vi "VI-Fill Temp Event Cluster.vi"(0 "VI in":refnum<vi>, 2 "Components":T1, 9 "Names":string[](array[string]), 11 "error in (no error)":errorcluster) -> (4 "VI out":refnum<vi>, 15 "error out":errorcluster)   [LabVIEW 2015]
uses:
  VI-Reg Event Components.ctl
  <vilib>/Utility/miscctls.llb/LVPointTypeDef.ctl
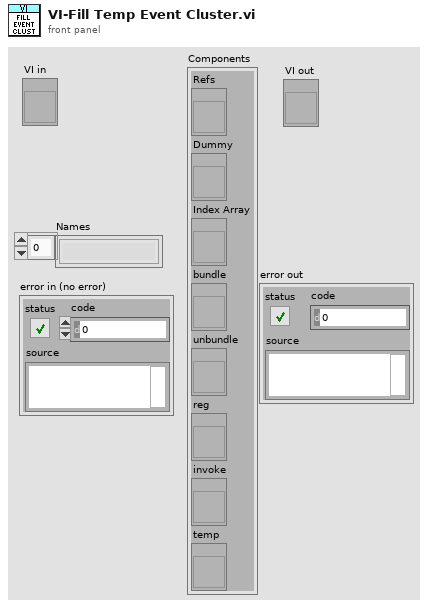
[diagram p1: front panel]
types:
  T1 = typedef "VI-Reg Event Components.ctl" = cluster{"Refs":refnum<vi>, "Dummy":refnum<vi>, "Index Array":refnum<vi>, "bundle":refnum<vi>, "unbundle":refnum<vi>, "reg":refnum<vi>, "invoke":refnum<vi>, "temp":refnum<vi>}
  T2 = typedef "LVPointTypeDef.ctl" = cluster{"Horizontal":i16, "Vertical":i16}
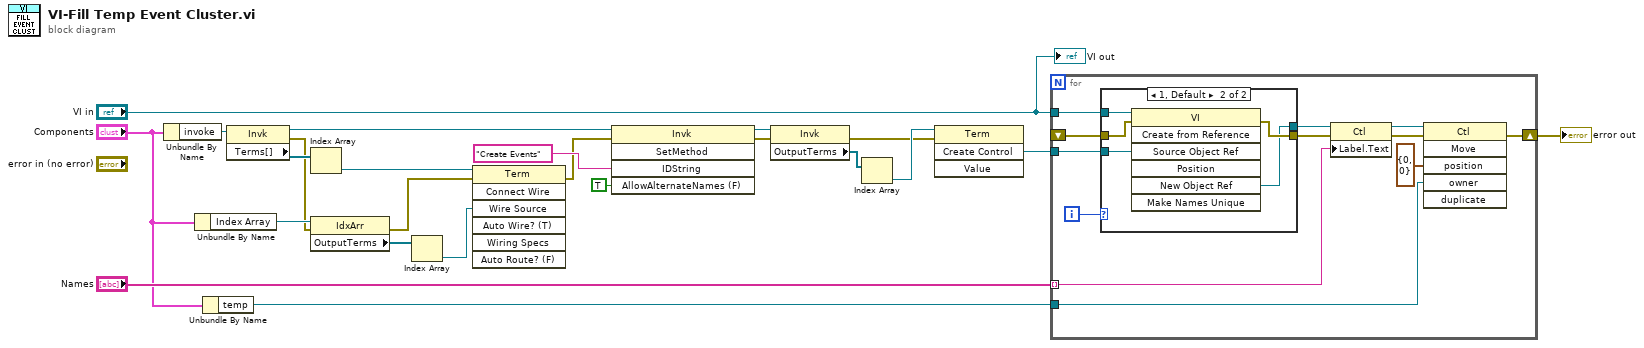
[diagram p0: block diagram]
diagram:
  n1 = Unbundle By Name("Components") -> ("invoke"=w1:refnum<vi>)
  n2 = Unbundle By Name("Components") -> ("Index Array"=w14:refnum<vi>)
  n3 = Unbundle By Name("Components") -> ("temp"=w23:refnum<vi>)
  n4 = property class="Invk"(reference=w1) -> (reference out=w5:refnum<vi>, error out=w8:errorcluster, "Terms[]"=w17:refnum<vi>[])  [unwired: 1 in]
  n5 = Index Array(array=w17) -> (element=w16:refnum<vi>)  [unwired: 1 in]
  n6 = property class="IdxArr"(reference=w14, error in=w8) -> (error out=w4:errorcluster, "OutputTerms"=w13:refnum<vi>[])  [unwired: 1 out]
  n7 = Index Array(array=w13) -> (element=w12:refnum<vi>)  [unwired: 1 in]
  n8 = invoke class="Term" method="Connect Wire"(reference=w16, error in=w4, "Wire Source"=w12) -> (error out=w3:errorcluster)  [unwired: 4 in, 6 out]
  n9 = invoke class="Invk" method="SetMethod"(reference=w5, error in=w3, "IDString"="Create Events" ("ID String"), "AllowAlternateNames (F)"=TRUE ("Allow Alternate Names? (F)")) -> (reference out=w10:refnum<vi>, error out=w9:errorcluster)  [unwired: 1 in, 3 out]
  n10 = property class="Invk"(reference=w10, error in=w9) -> (error out=w11:errorcluster, "OutputTerms"=w19:refnum<vi>[])  [unwired: 1 out]
  n11 = Index Array(array=w19) -> (element=w18:refnum<vi>)  [unwired: 1 in]
  n12 = invoke class="Term" method="Create Control"(reference=w18, error in=w11) -> ("Create Control"=w15:refnum<vi>)  [unwired: 2 in, 3 out]
  n13 = for {
    tunnel: w15 -> [w31]
    shift-right: [w34] -> w21
    shift-left: _ -> [w32]
    tunnel: "Names" -> [w28] mode=indexing
    tunnel: "VI in" -> [w33]
    tunnel: w23 -> [w24]
    i -> [w25]
    n14 = case shown="1, Default" w25 {
      tunnel: w33 -> [_ w42]
      tunnel: w32 -> [w36 w41]
      tunnel: w31 -> [w37 w40]
      tunnel: [w36 w39] -> w29
      tunnel: [w37 w38] -> w30
      frame 0 {
      }
      frame 1, Default {
        n15 = invoke class="VI" method="Create from Reference"(reference=w42, error in=w41, "Source Object Ref"=w40) -> (error out=w39:errorcluster, "New Object Ref"=w38:refnum<vi>)  [unwired: 4 in, 5 out]
      }
    }
    n16 = property class="Ctl"(reference=w30, error in=w29, "Label.Text"=w28) -> (reference out=w26:refnum<vi>, error out=w27:errorcluster)
    n17 = invoke class="Ctl" method="Move"(reference=w26, error in=w27, "position"=T2 {"Horizontal"=0, "Vertical"=0} ("Position"), "owner"=w24) -> (error out=w34:errorcluster)  [unwired: 2 in, 5 out]
  }
  "error out" <- w21
  "VI out" <- "VI in"
